vi "test Unsigned Integer Data Integrity.vi"(8 "error in (no error)":errorcluster, 11 "Data Manipulation Tests in":refnum<class "Data Manipulation Tests.lvclass">) -> (0 "error out":errorcluster, 3 "Data Manipulation Tests out":refnum<class "Data Manipulation Tests.lvclass">)   [LabVIEW 2017, in "Pointer Tests.lvlib" / "Data Manipulation Tests.lvclass"]
uses:
  Data Manipulation Tests.lvclass
  Source/Classes/Pointer/Public/New/New (1B).vi
  Source/Classes/Pointer/Public/Write/Write (0D U8).vi
  Source/Classes/Pointer/Public/New/New (2B).vi
  Source/Classes/Pointer/Public/Write/Write (0D U16).vi
  Source/Classes/Pointer/Public/New/New (4B).vi
  Source/Classes/Pointer/Public/Write/Write (0D U32).vi
  Source/Classes/Pointer/Public/New/New (8B).vi
  Source/Classes/Pointer/Public/Write/Write (0D U64).vi
  Source/Classes/Pointer/Public/Write/Write (1D U8).vi
  Source/Classes/Pointer/Public/Write/Write (1D U16).vi
  Source/Classes/Pointer/Public/Write/Write (1D U32).vi
  Source/Classes/Pointer/Public/Write/Write (1D U64).vi
  Source/Classes/Pointer/Pointer.lvclass
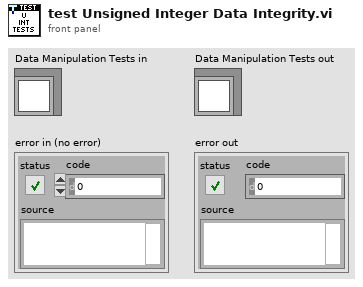
[diagram p1: front panel]
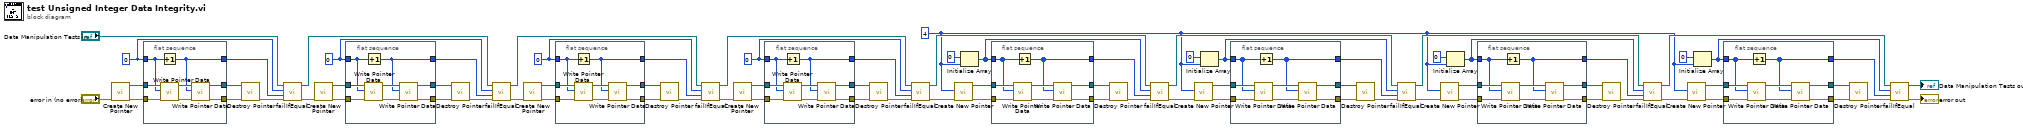
[diagram p0: block diagram]
diagram:
  w1 = u64 4 ("count (1)")
  w63 = u64 0 ("value")
  w74 = u32 0 ("value")
  w56 = u16 0 ("value")
  w45 = u8 0 ("value")
  n1 = call-poly "Create New Pointer.vi"("error in (no error)"="error in (no error)") -> ("error out"=w47:errorcluster, "Pointer"=w50:refnum<class "Pointer.lvclass">)  [unwired: 9 in]
  n2 = flat-sequence {
    tunnel: w50 -> [w87]
    tunnel: [w85] -> w49
    tunnel: [w84] -> w48
    tunnel: w47 -> [w82]
    tunnel: w45 -> [w81]
    tunnel: [w80] -> w44
    frame #0 {
      n3 = Increment(x=w81) -> (x+1=w80:u8)
      n4 = call-poly "Write Pointer Data.vi"("error in (no error)"=w82, "value"=w81, "Pointer in"=w87) -> ("error out"=w83:errorcluster, "Pointer out"=w86:refnum<class "Pointer.lvclass">)  [unwired: 5 in, 2 out]
      n5 = call-poly "Write Pointer Data.vi"("error in (no error)"=w83, "value"=w80, "Pointer in"=w86) -> ("error out"=w84:errorcluster, "Pointer out"=w85:refnum<class "Pointer.lvclass">)  [unwired: 5 in, 2 out]
    }
  }
  n6 = call "Destroy Pointer.vi"("error in (no error)"=w48, "Pointer in"=w49) -> ("error out"=w46:errorcluster)  [unwired: 8 in, 1 out]
  n7 = call-dynamic "failIfEqual.vi"("error in (no error)"=w46, "y"=w44, "x"=w45, "TestCase in"="Data Manipulation Tests in") -> ("error out"=w59:errorcluster, "TestCase out"=w58:refnum<class "Data Manipulation Tests.lvclass">)  [unwired: 6 in]
  n8 = call-poly "Create New Pointer.vi"("error in (no error)"=w59) -> ("error out"=w54:errorcluster, "Pointer"=w51:refnum<class "Pointer.lvclass">)  [unwired: 9 in]
  n9 = flat-sequence {
    tunnel: w51 -> [w95]
    tunnel: [w93] -> w52
    tunnel: [w92] -> w53
    tunnel: w54 -> [w90]
    tunnel: w56 -> [w89]
    tunnel: [w88] -> w57
    frame #0 {
      n10 = call-poly "Write Pointer Data.vi"("error in (no error)"=w90, "value"=w89, "Pointer in"=w95) -> ("error out"=w91:errorcluster, "Pointer out"=w94:refnum<class "Pointer.lvclass">)  [unwired: 5 in, 2 out]
      n11 = Increment(x=w89) -> (x+1=w88:u16)
      n12 = call-poly "Write Pointer Data.vi"("error in (no error)"=w91, "value"=w88, "Pointer in"=w94) -> ("error out"=w92:errorcluster, "Pointer out"=w93:refnum<class "Pointer.lvclass">)  [unwired: 5 in, 2 out]
    }
  }
  n13 = call "Destroy Pointer.vi"("error in (no error)"=w53, "Pointer in"=w52) -> ("error out"=w55:errorcluster)  [unwired: 8 in, 1 out]
  n14 = call-dynamic "failIfEqual.vi"("error in (no error)"=w55, "y"=w57, "x"=w56, "TestCase in"=w58) -> ("error out"=w77:errorcluster, "TestCase out"=w76:refnum<class "Data Manipulation Tests.lvclass">)  [unwired: 6 in]
  n15 = call-poly "Create New Pointer.vi"("error in (no error)"=w77) -> ("error out"=w72:errorcluster, "Pointer"=w69:refnum<class "Pointer.lvclass">)  [unwired: 9 in]
  n16 = flat-sequence {
    tunnel: w69 -> [w103]
    tunnel: [w101] -> w70
    tunnel: [w100] -> w71
    tunnel: w72 -> [w98]
    tunnel: w74 -> [w97]
    tunnel: [w96] -> w75
    frame #0 {
      n17 = call-poly "Write Pointer Data.vi"("error in (no error)"=w98, "value"=w97, "Pointer in"=w103) -> ("error out"=w99:errorcluster, "Pointer out"=w102:refnum<class "Pointer.lvclass">)  [unwired: 5 in, 2 out]
      n18 = Increment(x=w97) -> (x+1=w96:u32)
      n19 = call-poly "Write Pointer Data.vi"("error in (no error)"=w99, "value"=w96, "Pointer in"=w102) -> ("error out"=w100:errorcluster, "Pointer out"=w101:refnum<class "Pointer.lvclass">)  [unwired: 5 in, 2 out]
    }
  }
  n20 = call "Destroy Pointer.vi"("error in (no error)"=w71, "Pointer in"=w70) -> ("error out"=w73:errorcluster)  [unwired: 8 in, 1 out]
  n21 = call-dynamic "failIfEqual.vi"("error in (no error)"=w73, "y"=w75, "x"=w74, "TestCase in"=w76) -> ("error out"=w60:errorcluster, "TestCase out"=w61:refnum<class "Data Manipulation Tests.lvclass">)  [unwired: 6 in]
  n22 = call-poly "Create New Pointer.vi"("error in (no error)"=w60) -> ("error out"=w65:errorcluster, "Pointer"=w68:refnum<class "Pointer.lvclass">)  [unwired: 9 in]
  n23 = flat-sequence {
    tunnel: w68 -> [w111]
    tunnel: [w109] -> w67
    tunnel: [w108] -> w66
    tunnel: w65 -> [w106]
    tunnel: w63 -> [w105]
    tunnel: [w104] -> w62
    frame #0 {
      n24 = call-poly "Write Pointer Data.vi"("error in (no error)"=w106, "value"=w105, "Pointer in"=w111) -> ("error out"=w107:errorcluster, "Pointer out"=w110:refnum<class "Pointer.lvclass">)  [unwired: 5 in, 2 out]
      n25 = Increment(x=w105) -> (x+1=w104:u64)
      n26 = call-poly "Write Pointer Data.vi"("error in (no error)"=w107, "value"=w104, "Pointer in"=w110) -> ("error out"=w108:errorcluster, "Pointer out"=w109:refnum<class "Pointer.lvclass">)  [unwired: 5 in, 2 out]
    }
  }
  n27 = call "Destroy Pointer.vi"("error in (no error)"=w66, "Pointer in"=w67) -> ("error out"=w64:errorcluster)  [unwired: 8 in, 1 out]
  n28 = call-dynamic "failIfEqual.vi"("error in (no error)"=w64, "y"=w62, "x"=w63, "TestCase in"=w61) -> ("error out"=w12:errorcluster, "TestCase out"=w13:refnum<class "Data Manipulation Tests.lvclass">)  [unwired: 6 in]
  n29 = call-poly "Create New Pointer.vi"("error in (no error)"=w12, "count (1)"=w1) -> ("error out"=w41:errorcluster, "Pointer"=w38:refnum<class "Pointer.lvclass">)  [unwired: 8 in]
  n30 = Initialize Array(u8 0 ("value"), w1) -> (w8:u8[])
  n31 = flat-sequence {
    tunnel: w38 -> [w119]
    tunnel: [w117] -> w39
    tunnel: [w116] -> w40
    tunnel: w41 -> [w114]
    tunnel: w8 -> [w113]
    tunnel: [w112] -> w43
    frame #0 {
      n32 = call-poly "Write Pointer Data.vi"("error in (no error)"=w114, "buffer in"=w113, "Pointer in"=w119) -> ("error out"=w115:errorcluster, "Pointer out"=w118:refnum<class "Pointer.lvclass">)  [unwired: 5 in, 2 out]
      n33 = Increment(x=w113) -> (x+1=w112:u8[])
      n34 = call-poly "Write Pointer Data.vi"("error in (no error)"=w115, "buffer in"=w112, "Pointer in"=w118) -> ("error out"=w116:errorcluster, "Pointer out"=w117:refnum<class "Pointer.lvclass">)  [unwired: 5 in, 2 out]
    }
  }
  n35 = call "Destroy Pointer.vi"("error in (no error)"=w40, "Pointer in"=w39) -> ("error out"=w42:errorcluster)  [unwired: 8 in, 1 out]
  n36 = call-dynamic "failIfEqual.vi"("error in (no error)"=w42, "y"=w43, "x"=w8, "TestCase in"=w13) -> ("error out"=w30:errorcluster, "TestCase out"=w31:refnum<class "Data Manipulation Tests.lvclass">)  [unwired: 6 in]
  n37 = call-poly "Create New Pointer.vi"("error in (no error)"=w30, "count (1)"=w1) -> ("error out"=w34:errorcluster, "Pointer"=w37:refnum<class "Pointer.lvclass">)  [unwired: 8 in]
  n38 = Initialize Array(u16 0 ("value"), w1) -> (w6:u16[])
  n39 = flat-sequence {
    tunnel: w37 -> [w127]
    tunnel: [w125] -> w36
    tunnel: [w124] -> w35
    tunnel: w34 -> [w122]
    tunnel: w6 -> [w121]
    tunnel: [w120] -> w32
    frame #0 {
      n40 = call-poly "Write Pointer Data.vi"("error in (no error)"=w122, "buffer in"=w121, "Pointer in"=w127) -> ("error out"=w123:errorcluster, "Pointer out"=w126:refnum<class "Pointer.lvclass">)  [unwired: 5 in, 2 out]
      n41 = Increment(x=w121) -> (x+1=w120:u16[])
      n42 = call-poly "Write Pointer Data.vi"("error in (no error)"=w123, "buffer in"=w120, "Pointer in"=w126) -> ("error out"=w124:errorcluster, "Pointer out"=w125:refnum<class "Pointer.lvclass">)  [unwired: 5 in, 2 out]
    }
  }
  n43 = call "Destroy Pointer.vi"("error in (no error)"=w35, "Pointer in"=w36) -> ("error out"=w33:errorcluster)  [unwired: 8 in, 1 out]
  n44 = call-dynamic "failIfEqual.vi"("error in (no error)"=w33, "y"=w32, "x"=w6, "TestCase in"=w31) -> ("error out"=w14:errorcluster, "TestCase out"=w15:refnum<class "Data Manipulation Tests.lvclass">)  [unwired: 6 in]
  n45 = call-poly "Create New Pointer.vi"("error in (no error)"=w14, "count (1)"=w1) -> ("error out"=w18:errorcluster, "Pointer"=w21:refnum<class "Pointer.lvclass">)  [unwired: 8 in]
  n46 = Initialize Array(u32 0 ("value"), w1) -> (w4:u32[])
  n47 = flat-sequence {
    tunnel: w21 -> [w135]
    tunnel: [w133] -> w20
    tunnel: [w132] -> w19
    tunnel: w18 -> [w130]
    tunnel: w4 -> [w129]
    tunnel: [w128] -> w16
    frame #0 {
      n48 = call-poly "Write Pointer Data.vi"("error in (no error)"=w130, "buffer in"=w129, "Pointer in"=w135) -> ("error out"=w131:errorcluster, "Pointer out"=w134:refnum<class "Pointer.lvclass">)  [unwired: 5 in, 2 out]
      n49 = Increment(x=w129) -> (x+1=w128:u32[])
      n50 = call-poly "Write Pointer Data.vi"("error in (no error)"=w131, "buffer in"=w128, "Pointer in"=w134) -> ("error out"=w132:errorcluster, "Pointer out"=w133:refnum<class "Pointer.lvclass">)  [unwired: 5 in, 2 out]
    }
  }
  n51 = call "Destroy Pointer.vi"("error in (no error)"=w19, "Pointer in"=w20) -> ("error out"=w17:errorcluster)  [unwired: 8 in, 1 out]
  n52 = call-dynamic "failIfEqual.vi"("error in (no error)"=w17, "y"=w16, "x"=w4, "TestCase in"=w15) -> ("error out"=w29:errorcluster, "TestCase out"=w28:refnum<class "Data Manipulation Tests.lvclass">)  [unwired: 6 in]
  n53 = call-poly "Create New Pointer.vi"("error in (no error)"=w29, "count (1)"=w1) -> ("error out"=w25:errorcluster, "Pointer"=w22:refnum<class "Pointer.lvclass">)  [unwired: 8 in]
  n54 = Initialize Array(u64 0 ("value"), w1) -> (w2:u64[])
  n55 = flat-sequence {
    tunnel: w22 -> [w143]
    tunnel: [w141] -> w23
    tunnel: [w140] -> w24
    tunnel: w25 -> [w138]
    tunnel: w2 -> [w137]
    tunnel: [w136] -> w27
    frame #0 {
      n56 = call-poly "Write Pointer Data.vi"("error in (no error)"=w138, "buffer in"=w137, "Pointer in"=w143) -> ("error out"=w139:errorcluster, "Pointer out"=w142:refnum<class "Pointer.lvclass">)  [unwired: 5 in, 2 out]
      n57 = Increment(x=w137) -> (x+1=w136:u64[])
      n58 = call-poly "Write Pointer Data.vi"("error in (no error)"=w139, "buffer in"=w136, "Pointer in"=w142) -> ("error out"=w140:errorcluster, "Pointer out"=w141:refnum<class "Pointer.lvclass">)  [unwired: 5 in, 2 out]
    }
  }
  n59 = call "Destroy Pointer.vi"("error in (no error)"=w24, "Pointer in"=w23) -> ("error out"=w26:errorcluster)  [unwired: 8 in, 1 out]
  n60 = call-dynamic "failIfEqual.vi"("error in (no error)"=w26, "y"=w27, "x"=w2, "TestCase in"=w28) -> ("error out"=→"error out":errorcluster, "TestCase out"=→"Data Manipulation Tests out":refnum<class "Data Manipulation Tests.lvclass">)  [unwired: 6 in]
